vi "MultiChannelType_1D-Array-I8.vi"(9 "error in":errorcluster, 11 "Array in":i8[](array[numeric])) -> (1 "error out":errorcluster, 2 "MultiChannelType":u32, 3 "Array out":i8[](array[numeric]))   [LabVIEW 2020, in "OpenLvVision_OpenCv.lvlib"]
uses:
  OpenLvVision_OpenCv.lvlib
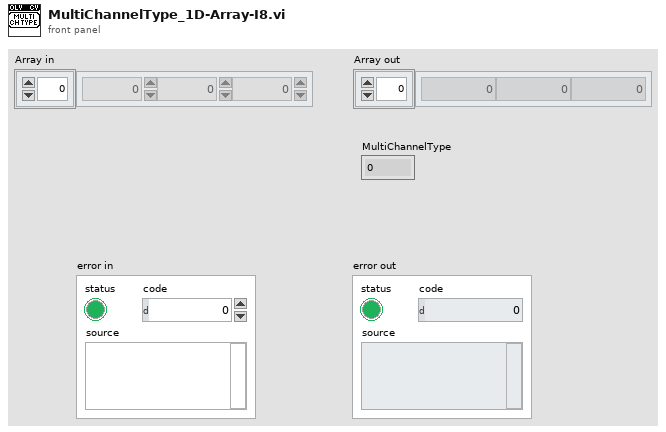
[diagram p1: front panel]
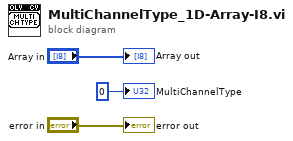
[diagram p0: block diagram]
diagram:
  "error out" <- "error in"
  "Array out" <- "Array in"
  "MultiChannelType" <- u32 0
